vi "HDF5_append-dataset-Test7vi.vi"() -> ()   [LabVIEW 2018]
uses:
  <vilib>/addons/h5labview2/file/H5F.lvlib
  <vilib>/addons/h5labview2/file/H5Fmode.ctl
  <vilib>/addons/h5labview2/dataset/H5D.lvlib
  HDF5/HDF5_ToneInfoClust.ctl
  <vilib>/addons/h5labview2/dataset/H5Dwrite.llb/H5Dwrite.xnode
  <vilib>/addons/h5labview2/space/H5S.lvlib
  <vilib>/addons/h5labview2/base/H5Equery.vi
  HDF5/lib_path_mod_20200519.vi
  <vilib>/addons/h5labview2/dataset/H5Dread.llb/H5Dread.xnode
  <vilib>/addons/h5labview2/group/H5G.lvlib
  <vilib>/addons/h5labview2/base/hid_t_renamed.ctl
panel:
  in  "Zoom":dbl[](array[numeric])
  out "Tone2":T1[](array[typedef])
  out "Tone1":T1[](array[typedef])
  out "ms/append":dbl
  out "timer (ms)":u32
  out "progress":i32(slide)=9999 scale=0.0..10.0
  in  "repetitions":i32=10
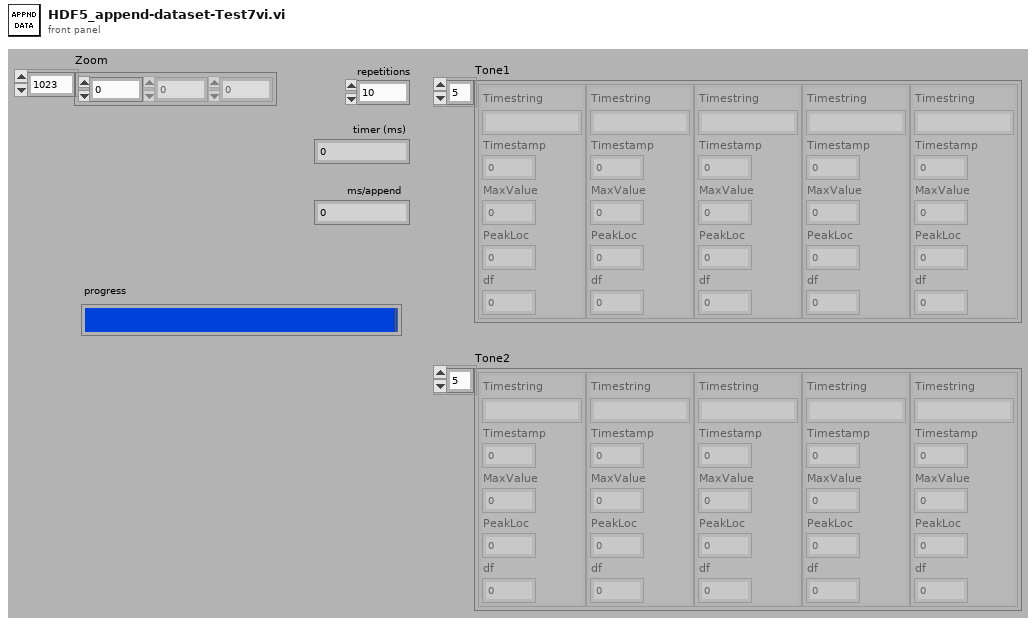
[diagram p1: front panel]
types:
  T1 = typedef "HDF5_ToneInfoClust.ctl" = cluster{"Timestring":string, "Timestamp":dbl, "MaxValue":dbl, "PeakLoc":dbl, "df":dbl}
  T2 = typedef "H5F.lvlib/H5Fmode.ctl" = enum16{"read-only", "read-write", "overwrite", "create new", "open or create"}
  T3 = typedef "HDF5_ToneInfoClust.ctl" = cluster{"Timestring":string, "Timestamp":timestamp, "MaxValue":dbl, "PeakLoc":dbl, "df":dbl}
  T4 = typedef "hid_t.ctl" = i32
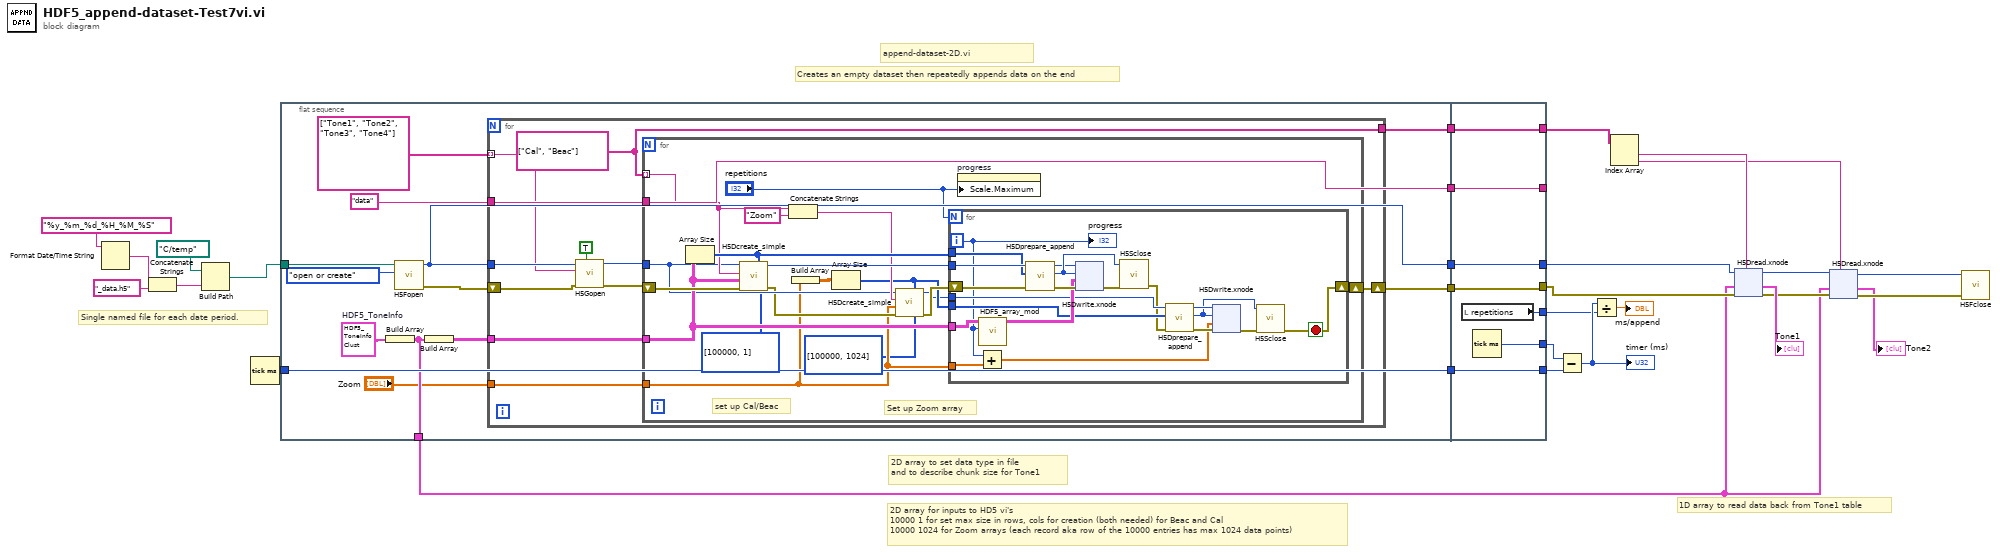
[diagram p0: block diagram]
diagram:
  # "2D array to set data type in file\nand to describe chunk size for Tone1"
  # "1D array to read data back from Tone1 table"
  # "2D array for inputs to HD5 vi's\n10000 1 for set max size in rows, cols for creation (both needed) for Beac and Cal\n10000 1024 for Zoom arrays (each record aka row of the 10000 entries has max 1024 data points)"
  # "Single named file for each date period."
  # "Creates an empty dataset then repeatedly appends data on the end"
  # "append-dataset-2D.vi"
  n1 = Format Date/Time String(time format string (%c)="%y_%m_%d_%H_%M_%S") -> (date/time string=w19:string)  [unwired: 2 in]
  n2 = Concatenate Strings(w19, "_data.h5" ("string")) -> (w21:string)
  n3 = Build Path(base path=path "C:/temp", name or relative path=w21) -> (appended path=w17:path)
  n4 = Tick Count (ms)() -> (millisecond timer value=w29:u32)
  n5 = flat-sequence {
    tunnel: w29 -> [w41]
    tunnel: [w41] -> w28
    tunnel: w17 -> [w40]
    tunnel: [w32] -> w15
    tunnel: [w37] -> w14
    tunnel: [w36] -> w2
    tunnel: [w35] -> w12
    tunnel: [w34] -> w10
    tunnel: w28 -> [w135]
    tunnel: [w136] -> w27
    tunnel: [w135] -> w26
    tunnel: [w134] -> w24
    tunnel: [w133] -> w16
    tunnel: w15 -> [w133]
    tunnel: [w132] -> _
    tunnel: w14 -> [w132]
    tunnel: [w131] -> w11
    tunnel: w12 -> [w131]
    tunnel: w10 -> [w130]
    tunnel: [w130] -> w8
    frame #0 {
      w39 = T3 {"Timestring"="Timestamp string goes here", "Timestamp"=timestamp(0 s since 1904-01-01), "MaxValue"=0.0, "PeakLoc"=0.0, "df"=0.0}  # HDF5_ToneInfo
      w37 = "data" ("name")
      n6 = Build Array(w39) -> (w36:T3[])
      n7 = call <vilib>:"H5Fopen.vi"("mode (read-only)"=H5Fmode."open or create" ("mode"), "path"=w40) -> ("error out"=w31:errorcluster, "ref out"=w32:T4)  [unwired: 8 in]
      n8 = Build Array(w36) -> (w38:T3[][])
      n9 = for {
        tunnel: w38 -> [w53]
        tunnel: w37 -> [w52]
        tunnel: [w50] -> w34
        tunnel: "Zoom" -> [w49]
        tunnel: w32 -> [w48]
        shift-right: [w51] -> w35
        shift-left: w31 -> [w44]
        tunnel: string[] ["Tone1", "Tone2", "Tone3", "Tone4"] -> [w43] mode=indexing
        w50 = string[] ["Cal", "Beac"]
        n10 = call <vilib>:"H5Gopen.vi"("create? (F)"=TRUE, "error in (no error)"=w44, "name"=w43, "ref in"=w48) -> ("error out"=w45:errorcluster, "group out"=w46:T4)  [unwired: 6 in]
        n11 = for {
          tunnel: w53 -> [w68]
          tunnel: w46 -> [w62]
          tunnel: w52 -> [_]
          shift-right: [w66] -> w51
          shift-left: w45 -> [w70]
          tunnel: w50 -> [w65] mode=indexing
          tunnel: w49 -> [w55]
          # "Set up Zoom array"
          # "set up Cal/Beac"
          n12 = Array Size(array=w68) -> (size(s)=w67:i32[])
          n13 = call <vilib>:"H5Dcreate_simple.vi"("max size"=u64[] [100000, 1], "chunk size"=w67, "error in (no error)"=w70, "type in"=w68, "name"=w65, "ref in"=w62) -> ("error out"=w59:errorcluster, "dset out"=w71:T4)  [unwired: 4 in]
          n14 = Concatenate Strings(w65, "Zoom" ("string")) -> (w63:string)
          n15 = Build Array(w55) -> (w61:dbl[][])
          n16 = Array Size(array=w61) -> (size(s)=w57:i32[])
          n17 = call <vilib>:"H5Dcreate_simple.vi"("max size"=u64[] [100000, 1024], "chunk size"=w57, "error in (no error)"=w59, "type in"=w55, "name"=w63, "ref in"=w62) -> ("error out"=w58:errorcluster, "dset out"=w56:T4)  [unwired: 4 in]
          n18 = for {
            N: "repetitions" -> [_]
            shift-right: [w75] -> w66
            shift-left: w58 -> [w88]
            tunnel: w67 -> [w89]
            tunnel: w71 -> [w90]
            tunnel: w68 -> [w84]
            tunnel: w57 -> [w82]
            tunnel: w56 -> [w81]
            tunnel: w55 -> [w73]
            i -> [w74]
            stop <- w75 stop-if-true
            n19 = Add(x=w74, y=w73) -> (x+y=w72:dbl[])
            n20 = call "HDF5_array_mod.vi"("delta"=w74, "Array in"=w84) -> ("Array out"=w83:T1[][])  [unwired: 9 in]
            n21 = call <vilib>:"H5Dprepare_append.vi"("error in (no error)"=w88, "append dims"=w89, "dset in"=w90) -> ("error out"=w91:errorcluster, "space out"=w86:T4, "dset out"=w85:T4)  [unwired: 5 in, 1 out]
            n22 = xnode "H5Dwrite.xnode"("error in (no error)"=w91, "data"=w83, "file space"=w86, "ref in"=w85) -> ("error out"=w87:errorcluster)  [unwired: 3 in, 2 out]
            n23 = call <vilib>:"H5Sclose.vi"("error in (no error)"=w87, "space in"=w86) -> ("error out"=w80:errorcluster)  [unwired: 9 in]
            n24 = call <vilib>:"H5Dprepare_append.vi"("error in (no error)"=w80, "append dims"=w82, "dset in"=w81) -> ("error out"=w77:errorcluster, "space out"=w78:T4, "dset out"=w79:T4)  [unwired: 5 in, 1 out]
            n25 = xnode "H5Dwrite.xnode"("error in (no error)"=w77, "data"=w72, "file space"=w78, "ref in"=w79) -> ("error out"=w76:errorcluster)  [unwired: 3 in, 2 out]
            n26 = call <vilib>:"H5Sclose.vi"("error in (no error)"=w76, "space in"=w78) -> ("error out"=w75:errorcluster)  [unwired: 9 in]
            "progress" <- w74
          }
          n27 = property on="progress" class="Slide (strict)"("Scale.Maximum"="repetitions") -> ()  [unwired: 2 in, 2 out]
        }
      }
    }
    frame #1 {
      n28 = local read "repetitions"() -> (w134:i32)
      n29 = Tick Count (ms)() -> (millisecond timer value=w136:u32)
    }
  }
  n30 = Subtract(x=w27, y=w26) -> (x-y=w25:u32)
  "timer (ms)" <- w25
  n31 = Divide(x=w25, y=w24) -> (x/y=→"ms/append":dbl)
  n32 = Index Array(array=w8) -> (element #1=w7:string, element #2=w6:string)  [unwired: 2 in]
  n33 = xnode "H5Dread.xnode"("dataset name (this)"=w7, "error in (no error)"=w11, "default"=w2, "ref in"=w16) -> ("error out"=w5:errorcluster, "data"=→"Tone1":T3[], "ref out"=w9:i32)  [unwired: 2 in, 1 out]
  n34 = xnode "H5Dread.xnode"("dataset name (this)"=w6, "error in (no error)"=w5, "default"=w2, "ref in"=w9) -> ("error out"=w3:errorcluster, "data"=→"Tone2":T3[], "ref out"=w4:i32)  [unwired: 2 in, 1 out]
  n35 = call <vilib>:"H5Fclose.vi"("error in (no error)"=w3, "ref"=w4) -> ()  [unwired: 9 in, 1 out]
